vi "Update Humidity Control Range.vi"(6 "RH":sgl, 8 "error in":errorcluster, 9 "Tcell":sgl, 10 "index":i32, 11 "cCRDS in":refnum<class "cCRDS.lvclass">=refnum) -> (0 "error out":errorcluster, 3 "cCRDS out":refnum<class "cCRDS.lvclass">)   [LabVIEW 2012, in "cCRDS.lvclass"]
uses:
  cCRDS.lvclass
  Reusable/General/Atmospheric/Atmospheric Library.lvlib
  Reusable/General/Temperature/Temperature.lvlib
  Reusable/Humidity Control/Base/Humidity Control.lvclass
  Reusable/Humidity Control/TEC/TEC Humidity Control.lvclass
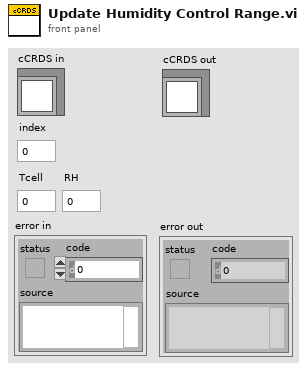
[diagram p1: front panel]
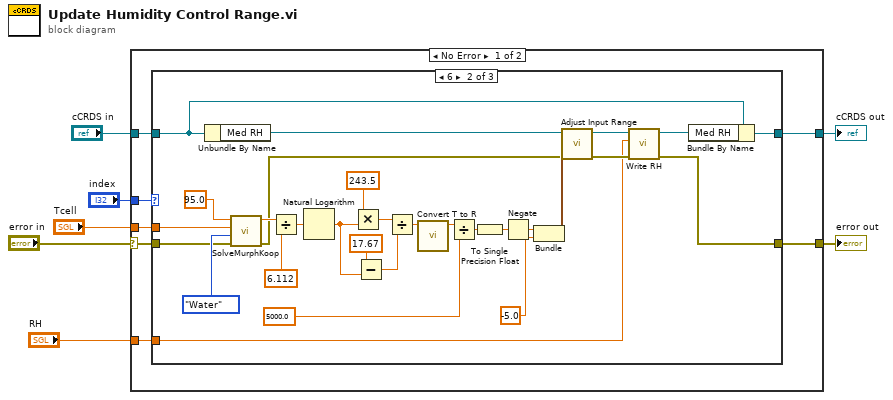
[diagram p0: block diagram]
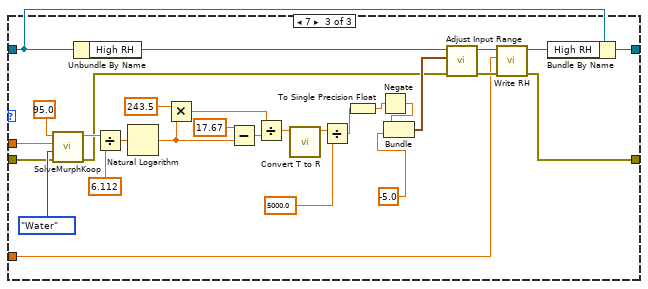
[diagram p3: hidden frame]
diagram:
  n1 = case shown="No Error" "error in" {
    selector: "error in" -> [w10 w76]
    tunnel: [w9 w76] -> w6
    tunnel: [w11 w75] -> w4
    tunnel: "cCRDS in" -> [w13 w75]
    tunnel: "index" -> [w14 _]
    tunnel: "Tcell" -> [w12 _]
    tunnel: "RH" -> [w8 _]
    frame No Error {
      n2 = case shown="6" w14 {
        tunnel: w13 -> [w16 w17 w57]
        tunnel: w12 -> [_ w28 w73]
        tunnel: [w16 w29 w56] -> w11
        tunnel: w10 -> [w15 w27 w55]
        tunnel: [w15 w20 w47] -> w9
        tunnel: w8 -> [_ w18 w46]
        frame 0, Default {
        }
        frame 6 {
          n3 = Unbundle By Name(w17) -> ("Med RH"=w35:refnum<class "TEC Humidity Control.lvclass">)
          n4 = call "SolveMurphKoop.vi"("Error In"=w27, "Type"=enum16{"Ice", "Water"}."Water", "T"=w28, "RH"=95.0) -> ("Error Out"=w26:errorcluster, "e"=w40:dbl)  [unwired: 4 in, 2 out]
          n5 = Divide(x=w40, y=6.112) -> (x/y=w39:dbl)
          n6 = Natural Logarithm(1:w39) -> (0:w38:dbl)
          n7 = Multiply(x=243.5, y=w38) -> (x*y=w37:dbl)
          n8 = Subtract(x=17.67, y=w38) -> (x-y=w36:dbl)
          n9 = Divide(x=w37, y=w36) -> (x/y=w34:dbl)
          n10 = call "Convert T to R.vi"("T"=w34) -> ("R"=w33:dbl)  [unwired: 10 in]
          n11 = Divide(x=w33, y=5000.0) -> (x/y=w31:dbl)
          n12 = To Single Precision Float(number=w31) -> (single precision float=w25:sgl)
          n13 = Negate(x=w25) -> (-x=w24:sgl)
          n14 = Bundle(w24, sgl -5.0) -> (w30:cluster{sgl, sgl})  [unwired: 1 in]
          n15 = call-dynamic "Adjust Input Range.vi"("error in"=w26, "Range Input"=w30, "Humidity Control in"=w35) -> ("error out"=w19:errorcluster, "Humidity Control out"=w22:refnum<class "TEC Humidity Control.lvclass">)  [unwired: 7 in]
          n16 = call "Write RH.vi"("error in (no error)"=w19, "RH"=w18, "Humidity Control in"=w22) -> ("error out"=w20:errorcluster, "Humidity Control out"=w21:refnum<class "TEC Humidity Control.lvclass">)  [unwired: 7 in]
          n17 = Bundle By Name(cluster=w17, "Med RH"=w21) -> (w29:refnum<class "cCRDS.lvclass">)
        }
        frame 7 {
          n18 = call "SolveMurphKoop.vi"("Error In"=w55, "Type"=enum16{"Ice", "Water"}."Water", "T"=w73, "RH"=95.0) -> ("Error Out"=w54:errorcluster, "e"=w68:dbl)  [unwired: 4 in, 2 out]
          n19 = Unbundle By Name(w57) -> ("High RH"=w63:refnum<class "TEC Humidity Control.lvclass">)
          n20 = Divide(x=w68, y=6.112) -> (x/y=w67:dbl)
          n21 = Natural Logarithm(1:w67) -> (0:w66:dbl)
          n22 = Multiply(x=243.5, y=w66) -> (x*y=w65:dbl)
          n23 = Subtract(x=17.67, y=w66) -> (x-y=w64:dbl)
          n24 = Divide(x=w65, y=w64) -> (x/y=w62:dbl)
          n25 = call "Convert T to R.vi"("T"=w62) -> ("R"=w61:dbl)  [unwired: 10 in]
          n26 = Divide(x=w61, y=5000.0) -> (x/y=w59:dbl)
          n27 = To Single Precision Float(number=w59) -> (single precision float=w53:sgl)
          n28 = Negate(x=w53) -> (-x=w52:sgl)
          n29 = Bundle(w52, sgl -5.0) -> (w58:cluster{sgl, sgl})  [unwired: 1 in]
          n30 = call-dynamic "Adjust Input Range.vi"("error in"=w54, "Range Input"=w58, "Humidity Control in"=w63) -> ("error out"=w48:errorcluster, "Humidity Control out"=w50:refnum<class "TEC Humidity Control.lvclass">)  [unwired: 7 in]
          n31 = call "Write RH.vi"("error in (no error)"=w48, "RH"=w46, "Humidity Control in"=w50) -> ("error out"=w47:errorcluster, "Humidity Control out"=w49:refnum<class "TEC Humidity Control.lvclass">)  [unwired: 7 in]
          n32 = Bundle By Name(cluster=w57, "High RH"=w49) -> (w56:refnum<class "cCRDS.lvclass">)
        }
      }
    }
    frame Error {
    }
  }
  "error out" <- w6
  "cCRDS out" <- w4
